vi "Configure Measurement (Frequency).vi"(7 "Frequency Resolution (1 Hz)":dbl=1.0, 8 "error in (no error)":errorcluster, 9 "Frequency Estimate (10E+6 Hz)":dbl=10000000.0 format="%^#_6g", 10 "Channel (1:Channel 1)":i32(ring)=1 items=["Channel 1"=1, "Channel 2"=2, "Channel 3"=3], 11 "VISA resource name":refnum<visa-resource-name>) -> (0 "error out":errorcluster, 3 "VISA resource name out":refnum<visa-resource-name>)   [LabVIEW 2024, in "Agilent 532XX Series.lvlib"]
doc: "Configures the settings required for a Frequency measurement."
uses:
  Agilent 532XX Series.lvlib
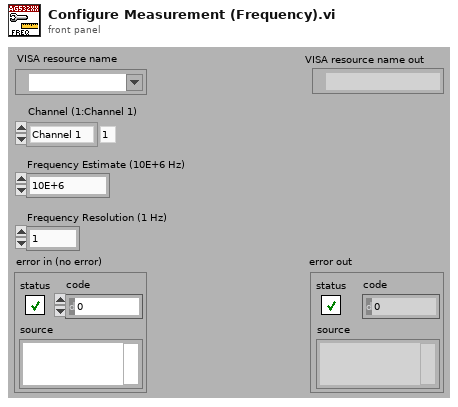
[diagram p1: front panel]
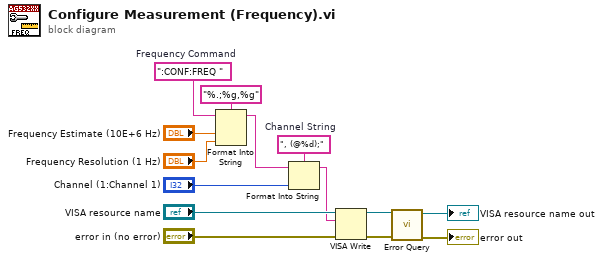
[diagram p0: block diagram]
diagram:
  w10 = ", (@%d);"  # Channel String
  w2 = ":CONF:FREQ "  # Frequency Command
  n1 = Format Into String(format string="%.;%g,%g", initial string=w2, "Frequency Estimate (10E+6 Hz)", "Frequency Resolution (1 Hz)") -> (resulting string=w3:string)  [unwired: 1 in, 1 out]
  n2 = Format Into String(format string=w10, initial string=w3, "Channel (1:Channel 1)") -> (resulting string=w4:string)  [unwired: 1 in, 1 out]
  n3 = VISA Write(VISA resource name="VISA resource name", write buffer=w4, error in (no error)="error in (no error)") -> (VISA resource name out=w9:refnum<visa-resource-name>, error out=w7:errorcluster)  [unwired: 1 out]
  n4 = call "Error Query.vi"("error in (no error)"=w7, "VISA resource name"=w9) -> ("error out"=→"error out":errorcluster, "VISA resource name out"=→"VISA resource name out":refnum<visa-resource-name>)  [unwired: 8 out]
